vi "摆角通道创建-子.vi"() -> (0 "error out":errorcluster caption="错误输出", 1 "task out":refnum<k21> caption="任务输出")   [LabVIEW 2015]
uses:
  <vilib>/DAQmx/create/channels.llb/DAQmx Create Channel (CI-Count Edges).vi
  <resource>/objmgr/daqmx.rc
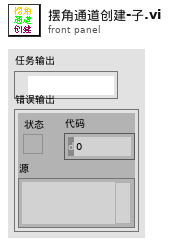
[diagram p1: front panel]
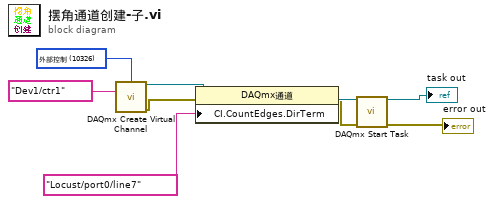
[diagram p0: block diagram]
diagram:
  w9 = 10326 items=["升值计数"=10128, "减值计数"=10124, "外部控制"=10326] ("count direction")
  n1 = call-poly <vilib>:"DAQmx Create Virtual Channel.vi"("count direction"=w9, "counter"=tag "Dev1/ctr1") -> ("task out"=w7:refnum<k21>, "error out"=w4:errorcluster)  [unwired: 12 in]
  n2 = property class="DAQmx通道"(reference=w7, error in=w4, "CI.CountEdges.DirTerm"=tag "Locust/port0/line7" ("CI.CountEdges.Term")) -> (reference out=w6:refnum<k21>, error out=w5:errorcluster)
  n3 = call <vilib>:"DAQmx Start Task.vi"("task/channels in"=w6, "error in"=w5) -> ("task out"=→"task out":refnum<k21>, "error out"=→"error out":errorcluster)  [unwired: 12 in]
